vi "Drive Logic.vi"(6 "dt (s)":dbl, 8 "error in (no error)":errorcluster, 10 "Drive Inputs":T3) -> (0 "error out":errorcluster, 2 "Drive Outputs":T2)   [LabVIEW 2014]
uses:
  Drive Input Data.ctl
  Drive Output Data.ctl
  Utilities/Ramp.vi
  <vilib>/Rock Robotics/Network Tables/SD Read Boolean.vi
  <vilib>/Rock Robotics/Network Tables/SD Read Number.vi
panel:
  in  "Strafe Deadzone":dbl=0.15 format="%#_13g"
  in  "Rotation Deadzone":dbl=0.045 format="%#_13g"
  in  "Half Drive Scaling":dbl=0.5 format="%#_13g"
  in  "Throttle Deadzone":dbl=0.15 format="%#_13g"
  in  "Gyro PID gains":T1={"proportional gain (Kc)"=-0.05, "integral time (Ti, min)"=0.0, "derivative time (Td, min)"=0.0} {"derivative time (Td, min)" format="%.3f"; "integral time (Ti, min)" format="%.3f"; "proportional gain (Kc)" format="%.3f"}
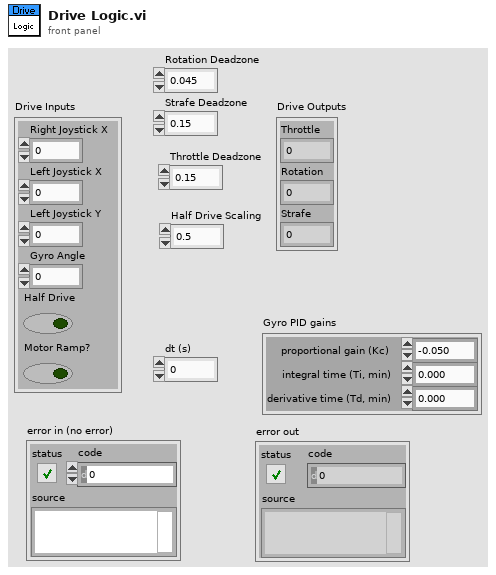
[diagram p1: front panel]
types:
  T1 = cluster{"proportional gain (Kc)":dbl, "integral time (Ti, min)":dbl, "derivative time (Td, min)":dbl}
  T2 = typedef "Drive Output Data.ctl" = cluster{"Throttle":dbl, "Rotation":dbl, "Strafe":dbl}
  T3 = typedef "Drive Input Data.ctl" = cluster{"Right Joystick X":dbl, "Left Joystick X":dbl, "Left Joystick Y":dbl, "Gyro Angle":dbl, "Half Drive":bool, "Motor Ramp?":bool}
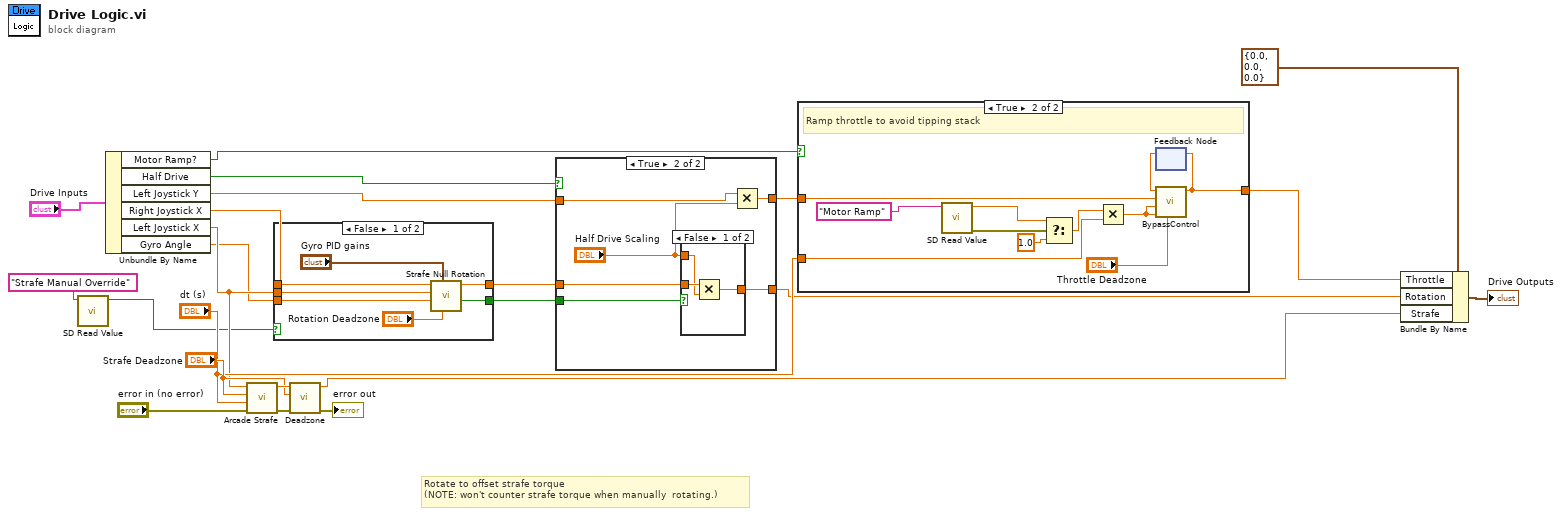
[diagram p0: block diagram]
diagram:
  # "Rotate to offset strafe torque\n(NOTE: won't counter strafe torque when manually  rotating.)"
  n1 = call-poly <vilib>:"SD Read Value.vi"("Name"="Strafe Manual Override") -> ("Boolean"=w3:bool)  [unwired: 8 in, 2 out]
  n2 = Unbundle By Name("Drive Inputs") -> ("Motor Ramp?"=w12:bool, "Half Drive"=w15:bool, "Left Joystick Y"=w16:dbl, "Right Joystick X"=w5:dbl, "Left Joystick X"=w8:dbl, "Gyro Angle"=w4:dbl)
  n3 = call "Arcade Strafe.vi"("error in"="error in (no error)", "dt (s)"="dt (s)", "Deadzone"="Strafe Deadzone", "Left Joystick X"=w8) -> ("error out"=w20:errorcluster, "Strafe Output"=w18:dbl)  [unwired: 6 in]
  n4 = case shown="False" w3 {
    tunnel: w5 -> [w27 w31]
    tunnel: [w29 w31] -> w7
    tunnel: [w30 _] -> w6
    tunnel: w4 -> [w28 _]
    tunnel: w8 -> [w26 _]
    frame False {
      n5 = call "Strafe Null Rotation.vi"("Deadzone"="Rotation Deadzone", "Gyro gains"="Gyro PID gains", "Gyro Angle"=w28, "Strafe (Left Joystick X)"=w26, "Rotation (Right Joystick X)"=w27) -> ("In deadzone?"=w30:bool, "Rotation"=w29:dbl)  [unwired: 4 in, 1 out]
    }
    frame True {
    }
  }
  n6 = call "Deadzone.vi"("error in (no error)"=w20, "Deadzone"="Strafe Deadzone", "Input"=w18) -> ("error out"=→"error out":errorcluster, "Output"=w9:dbl)  [unwired: 6 in, 1 out]
  n7 = case shown="True" w15 {
    tunnel: w16 -> [w33 w39]
    tunnel: w7 -> [w32 w38]
    tunnel: [w33 w36] -> w14
    tunnel: [w32 w35] -> w11
    tunnel: w6 -> [_ w34]
    frame False {
    }
    frame True {
      n8 = case shown="False" w34 {
        tunnel: w38 -> [w42 w43]
        tunnel: "Half Drive Scaling" -> [w41 _]
        tunnel: [w40 w43] -> w35
        frame False {
          n9 = Multiply(x=w42, y=w41) -> (x*y=w40:dbl)
        }
        frame True {
        }
      }
      n10 = Multiply(x=w39, y="Half Drive Scaling") -> (x*y=w36:dbl)
    }
  }
  n11 = case shown="True" w12 {
    tunnel: [w44 w47] -> w1
    tunnel: w14 -> [w44 w45]
    tunnel: "dt (s)" -> [_ w46]
    frame False {
      # "Pass through throttle"
    }
    frame True {
      # "Ramp throttle to avoid tipping stack"
      n12 = call-poly <vilib>:"SD Read Value.vi"("Name"="Motor Ramp") -> ("error out"=w50:errorcluster, "Numeric"=w51:dbl)  [unwired: 8 in, 1 out]
      n13 = Select(t=w51, s=w50, f=1.0 ("t")) -> (s? t:f=w54:dbl)
      n14 = Multiply(x=w54, y=w46) -> (x*y=w55:dbl)
      n15 = feedback #1() -> (w53:dbl)  [unwired: 1 in]
      n16 = call "BypassControl.vi"("Cutoff"="Throttle Deadzone", "MaxMotorChangeForward"=w55, "MaxMotorChangeBackward"=w55, "Current Input"=w45, "Previous Input"=w53) -> ("SetMotor"=w47:dbl)  [unwired: 5 in, 1 out]
      n17 = feedback-in #1(w47) -> ()
    }
  }
  n18 = Bundle By Name(cluster=T2 {"Throttle"=0.0, "Rotation"=0.0, "Strafe"=0.0} ("Drive Outputs"), "Throttle"=w1, "Rotation"=w11, "Strafe"=w9) -> (→"Drive Outputs":T2)
